vi "focusKnob.vi"() -> ()   [LabVIEW 2017]
panel:
  in  "position (10^-4 m)":i32=-1
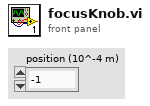
[diagram p1: front panel]
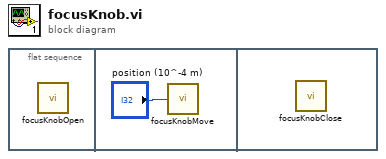
[diagram p0: block diagram]
diagram:
  n1 = flat-sequence {
    frame #0 {
      n2 = call "focusKnobOpen.vi"() -> ()  [unwired: 12 in]
    }
    frame #1 {
      n3 = call "focusKnobMove.vi"("position (10^-4 m)"="position (10^-4 m)") -> ()  [unwired: 1 in]
    }
    frame #2 {
      n4 = call "focusKnobClose.vi"() -> ()  [unwired: 12 in]
    }
  }
